vi "D2SParser - Private - Function - Read Character Status.vi"(8 "error in (no error)":errorcluster, 11 "D2SParser in":refnum<class "D2SParser.lvclass">) -> (0 "error out":errorcluster, 3 "D2SParser out":refnum<class "D2SParser.lvclass">)   [LabVIEW 2015, in "D2SParser.lvclass"]
uses:
  D2SParser.lvclass
  D2SParser.lvclass/D2SParser.ctl
  D2Character/D2Character.lvclass/D2Character.ctl
  D2Character/D2Character - Accessors - Set Status.vi
  D2SParser - Private - Helper - Read Byte.vi
  D2Character/D2Character.lvclass
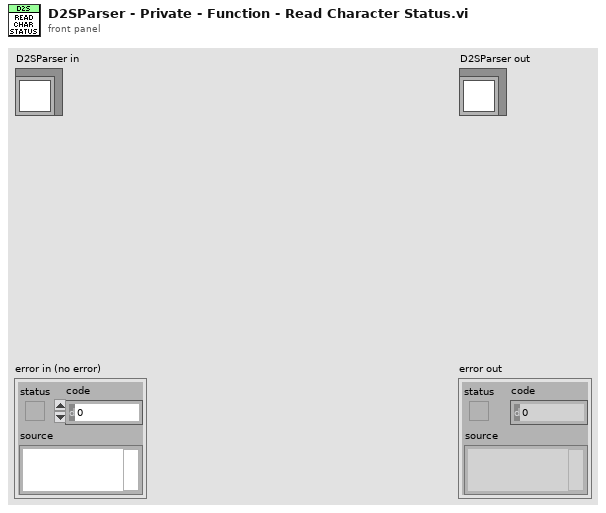
[diagram p1: front panel]
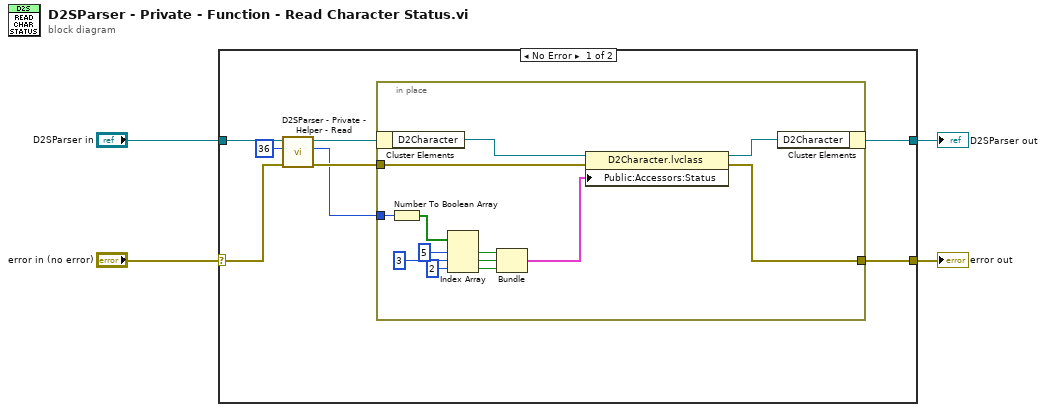
[diagram p0: block diagram]
diagram:
  n1 = case shown="No Error" "error in (no error)" {
    selector: "error in (no error)" -> [w11 w27]
    tunnel: [w8 w27] -> w3
    tunnel: [w7 w26] -> w1
    tunnel: "D2SParser in" -> [w12 w26]
    frame No Error {
      n2 = call-poly "D2SParser - Private - Helper - Read.vi"("error in (no error)"=w11, "Position"=i64 36, "D2SParser in"=w12) -> ("error out"=w9:errorcluster, "byte"=w5:u8, "D2SParser out"=w10:refnum<class "D2SParser.lvclass">)  [unwired: 6 in]
      n3 = in-place {
        in-place-border: w9 -> [w23]
        in-place-border: [w22] -> w8
        in-place-border: w5 -> [w21]
        n4 = in-place-cluster #1(w10) -> ("D2Character"=w25:refnum<class "D2Character.lvclass">)
        n5 = Number To Boolean Array(number=w21) -> (Boolean array=w20:bool[])
        n6 = Index Array(array=w20, index #1=5 ("index"), index #2=3 ("index"), index #3=2 ("index")) -> (element #1=w14:bool, element #2=w16:bool, element #3=w15:bool)
        n7 = Bundle(w14, w16, w15) -> (w13:cluster{bool, bool, bool})  [unwired: 1 in]
        n8 = property class="D2Character.lvclass"(reference=w25, error in=w23, "Public:Accessors:Status"=w13) -> (reference out=w24:refnum<class "D2Character.lvclass">, error out=w22:errorcluster)
        n9 = in-place-cluster #1("D2Character"=w24) -> (w7:refnum<class "D2SParser.lvclass">)
      }
    }
    frame Error {
    }
  }
  "error out" <- w3
  "D2SParser out" <- w1
